vi "AddEdge.vi"(6 "edgeSpec":string, 8 "error in (no error)":errorcluster, 9 "Target Port":refnum<class "FSM.Port.lvclass">, 10 "Source Port":refnum<class "FSM.Port.lvclass">, 11 "FSM in":refnum<class "FSM.Graph.lvclass">) -> (0 "error out":errorcluster, 2 "New Edge":refnum<class "FSM.Edge.lvclass">, 3 "FSM out":refnum<class "FSM.Graph.lvclass">)   [LabVIEW 2015, in "FSM.Graph.lvclass"]
uses:
  FSM.Graph.lvclass
  FSM.Port/FSM.Port.lvclass
  FSM.Edge/FSM.Edge.lvclass
  FSM.Graph.lvclass/FSM.Graph.ctl
  FSM.Port/FSM.Port.lvclass/FSM.Port.ctl
  FSM.Node/FSM.Node.lvclass/FSM.Node.ctl
  FSM.Port/Read belongsTo.vi
  FSM.Node/Read Shape.vi
  FSM.Node/FSM.Node.lvclass
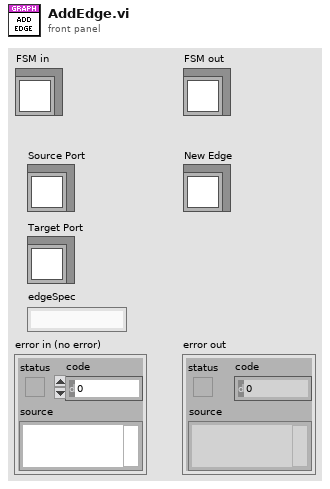
[diagram p1: front panel]
types:
  T1 = typedef "FSM.Node.lvclass/Shape.ctl" = enum16{"Default", "Start", "Action", "End"}
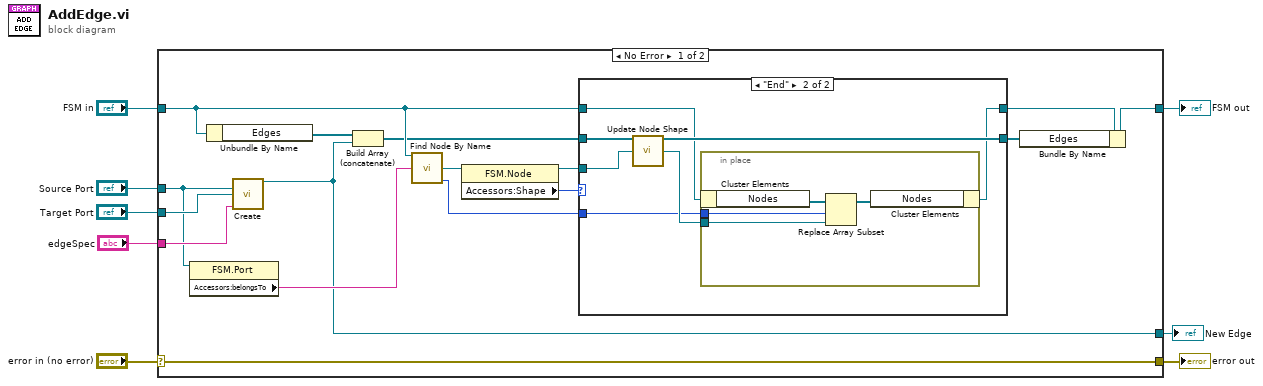
[diagram p0: block diagram]
diagram:
  n1 = case shown="No Error" "error in (no error)" {
    selector: "error in (no error)" -> [w24 w39]
    tunnel: [w24 w39] -> w7
    tunnel: [w11 w38] -> w5
    tunnel: "FSM in" -> [w14 w38]
    tunnel: "Target Port" -> [w22 _]
    tunnel: "Source Port" -> [w20 _]
    tunnel: "edgeSpec" -> [w21 _]
    tunnel: [w9 _] -> w1
    frame No Error {
      n2 = property class="FSM.Port"(reference=w20) -> ("Accessors:belongsTo"=w19:string)  [unwired: 1 in, 2 out]
      n3 = Unbundle By Name(w14) -> ("Edges"=w23:refnum<class "FSM.Edge.lvclass">[])
      n4 = call "Create.vi"("Source Port"=w20, "Target Port"=w22, "edgeSpec"=w21) -> ("New Edge"=w9:refnum<class "FSM.Edge.lvclass">)  [unwired: 12 in]
      n5 = Build Array (concatenate)(w23, w9) -> (w13:refnum<class "FSM.Edge.lvclass">[])
      n6 = call "Find Node By Name.vi"("FSM.Graph"=w14, "Name"=w19) -> ("Node"=w18:refnum<class "FSM.Node.lvclass">, "index"=w15:i32)  [unwired: 12 in]
      n7 = property class="FSM.Node"(reference=w18) -> (reference out=w16:refnum<class "FSM.Node.lvclass">, "Accessors:Shape"=w17:T1)  [unwired: 1 in, 1 out]
      n8 = case shown="\"End\"" w17 {
        tunnel: w16 -> [_ w32]
        tunnel: w15 -> [_ w28]
        tunnel: [w26 w27] -> w12
        tunnel: w14 -> [w26 w30]
        tunnel: w13 -> [w25 w33]
        tunnel: [w25 w31] -> w10
        frame "Default", Default {
        }
        frame "End" {
          n9 = call "Update Node Shape.vi"("Edges"=w33, "FSM.Node in"=w32) -> ("Edges Out"=w31:refnum<class "FSM.Edge.lvclass">[], "FSM.Node out"=w29:refnum<class "FSM.Node.lvclass">)  [unwired: 12 in]
          n10 = in-place {
            in-place-border: w29 -> [w35]
            in-place-border: w28 -> [w34]
            n11 = in-place-cluster #1(w30) -> ("Nodes"=w37:refnum<class "FSM.Node.lvclass">[])
            n12 = Replace Array Subset(array=w37, new element=w35, index=w34) -> (w36:refnum<class "FSM.Node.lvclass">[])
            n13 = in-place-cluster #1("Nodes"=w36) -> (w27:refnum<class "FSM.Graph.lvclass">)
          }
        }
      }
      n14 = Bundle By Name(cluster=w12, "Edges"=w10) -> (w11:refnum<class "FSM.Graph.lvclass">)
    }
    frame Error {
    }
  }
  "error out" <- w7
  "FSM out" <- w5
  "New Edge" <- w1
